vi "FTW-Actor-UserDefinedTraceEvent.vi"(0 "Event Type":string, 5 "Event Data":string, 11 "Error to Log":errorcluster, 12 "trace integer":i32) -> ()   [LabVIEW 2015]
uses:
  EventLogger/FTW-Logger.lvclass
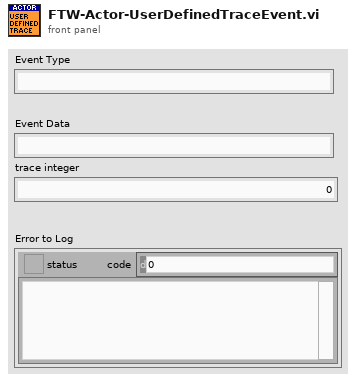
[diagram p1: front panel]
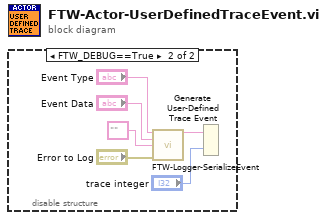
[diagram p0: block diagram]
diagram:
  n1 = disable-structure shown="FTW_DEBUG==True" {
    frame condition #0 (active) {
    }
    frame condition #1 {
      n2 = call "FTW-Logger-SerializeEvent.vi"("Event Type"="Event Type", "Event Data"="Event Data", "Source (unwired for call chain, Empty to omit)"="" ("empty string"), "Error to Log"="Error to Log") -> ("Serialized Event"=w6:string)  [unwired: 11 in]
      n3 = Generate User-Defined Trace Event(1:"trace integer", 2:w6) -> ()
    }
  }
